vi "Color_Sensor.vi"(11 "PhoenixMotorControlDevRef":T1={"DeviceStatus"={"status"=FALSE, "code"=0, "source"=""}, "Type"=enum."PWM", "PWM"={"PWM Channel"=enum."PWM 1", "DeadBand"={"Name"="", "maxPositivePwm"=0, "minPositivePwm"=0, "centerPwm"=0, "maxNegativePwm"=0, "minNegativePwm"=0, "angularRange"=0}}, "CAN"={"Device Number"=0, "SetOutput VI Ref"=variant(enum8{"Percent VBus", "Current", "Speed", "Position", "Voltage"} enum."Percent VBus"), "GetOutput VI Ref"=variant(refnum<k1> refnum), "Enable VI Ref"=variant(dbl 12.0), "Disable VI Ref"=variant(enum8{"Percent VBus", "Speed", "Position", "Slave", "Unchanged / Invalid", "Voltage Compensation", "Current", "Motion Profile"} enum."Percent VBus"), "Data"=variant}, "Invert"=FALSE, "DIO PWM"={"PWM \"Enable\" Channel"=enum."Invalid", "DIOChannel"=enum."Invalid", "PWM Rate"=0.0}}) -> ()   [LabVIEW 2019]
uses:
  <vilib>/Rock Robotics/WPI/MotorControl/WPI_MotorControlDeviceRef.ctl
  <vilib>/Rock Robotics/WPI/MotorControl/WPI_MotorControlType.ctl
  <vilib>/Rock Robotics/SystemInterfaces/DIO/FPGA_DIOPWMChannel.ctl
  <vilib>/Rock Robotics/WPI/PWM/WPI_PWMDeadband.ctl
  <vilib>/Rock Robotics/SystemInterfaces/DIO/FPGA_DIOChannel.ctl
  <vilib>/Rock Robotics/WPI/ThirdParty/Phoenix-LabVIEW/Motor Controller/Controls/CTRE_Phoenix_MotorControl_ControlMode.ctl
panel:
  out "Color Match? 2":bool
  out "Matched Color Name 2":string
  out "Match Confidence 2":dbl
  out "Measured Color 2":cluster{"R":dbl, "G":dbl, "B":dbl}
  out "error out 2":errorcluster
  out "Proximity 2":u16(graph)
  out "Color 2":u32(colorbox)
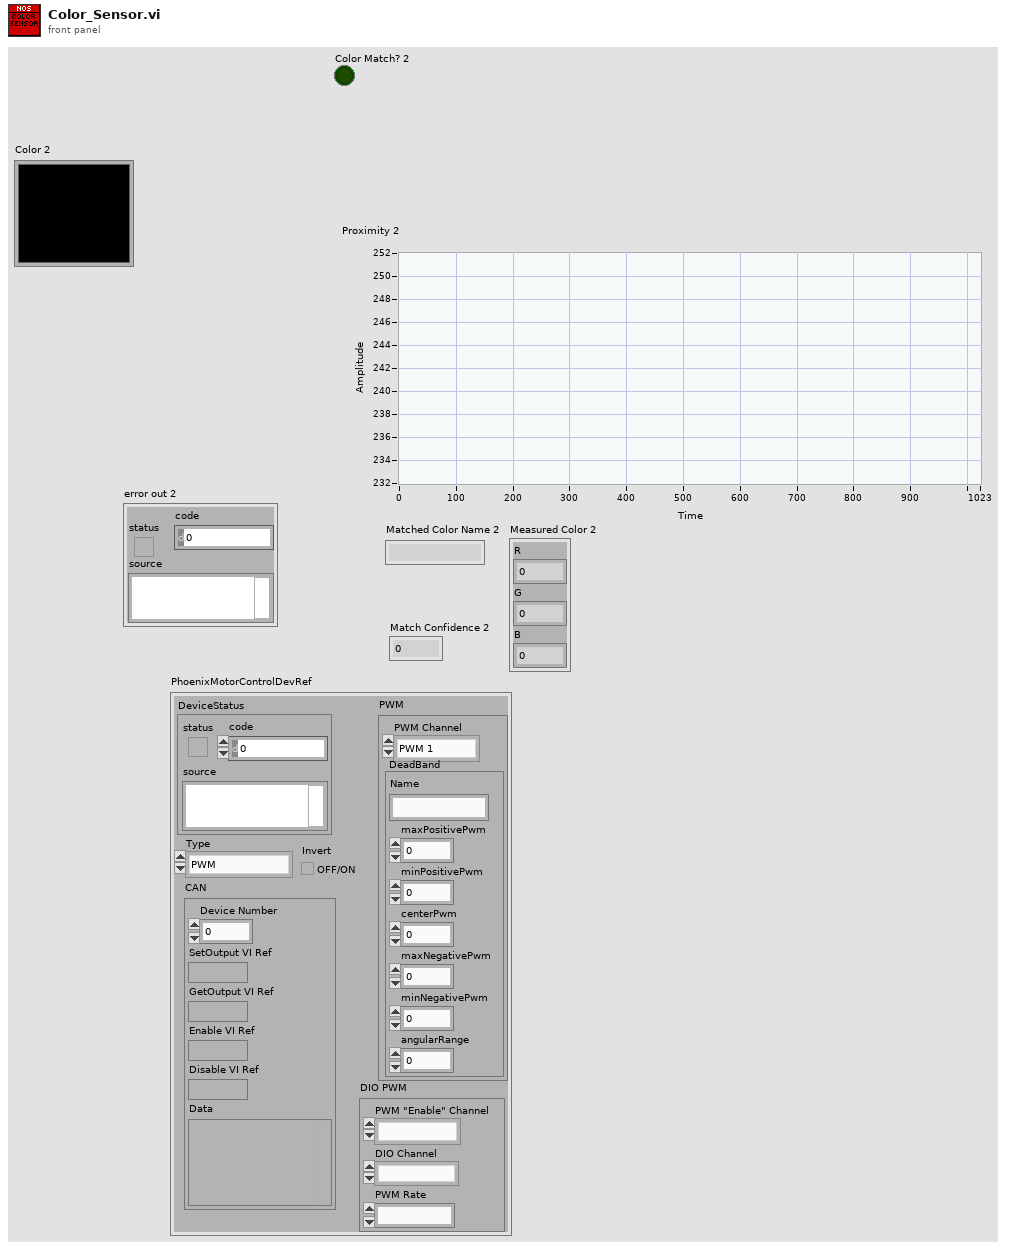
[diagram p1: front panel]
types:
  T1 = typedef "WPI_MotorControlDeviceRef.ctl" = cluster{"DeviceStatus":errorcluster, "Type":T2, "PWM":cluster{"PWM Channel":T3, "DeadBand":T4}, "CAN":cluster{"Device Number":u8, "SetOutput VI Ref":variant, "GetOutput VI Ref":variant, "Enable VI Ref":variant, "Disable VI Ref":variant, "Data":variant}, "Invert":bool, "DIO PWM":cluster{"PWM \"Enable\" Channel":T3, "DIOChannel":T5, "PWM Rate":dbl}}
  T2 = typedef "WPI_MotorControlType.ctl" = enum16{"PWM", "CAN", "DIO PWM"}
  T3 = typedef "FPGA_DIOPWMChannel.ctl" = enum8{"PWM 0", "PWM 1", "PWM 2", "PWM 3", "PWM 4", "PWM 5", "PWM 6", "PWM 7", "PWM 8", "PWM 9", "PWM MXP 0", "PWM MXP 1", "PWM MXP 2", "PWM MXP 3", "PWM MXP 4", "PWM MXP 5", "PWM MXP 6", "PWM MXP 7", "PWM MXP 8", "PWM MXP 9", "Invalid"}
  T4 = typedef "WPI_PWMDeadband.ctl" = cluster{"Name":string, "maxPositivePwm":i32, "minPositivePwm":i32, "centerPwm":i32, "maxNegativePwm":i32, "minNegativePwm":i32, "angularRange":u16}
  T5 = typedef "FPGA_DIOChannel.ctl" = enum8{"DIO 0", "DIO 1", "DIO 2", "DIO 3", "DIO 4", "DIO 5", "DIO 6", "DIO 7", "DIO 8", "DIO 9", "DIO MXP 0", "DIO MXP 1", "DIO MXP 2", "DIO MXP 3", "DIO MXP 4", "DIO MXP 5", "DIO MXP 6", "DIO MXP 7", "DIO MXP 8", "DIO MXP 9", "DIO MXP 10", "DIO MXP 11", "DIO MXP 12", "DIO MXP 13", "DIO MXP 14", "DIO MXP 15", "SPI Port CS1", "SPI Port CS2", "SPI Port CS3", "SPI Port MISO", "SPI Port MOSI", "Invalid"}
  T6 = typedef "CTRE_Phoenix_MotorControl_ControlMode.ctl" = u16
  T7 = typedef "Color Sensor V3 DevRef.ctl" = cluster{"I2CDevRef":T8}
  T8 = typedef "WPI_I2CDevRef.ctl" = cluster{"DevStatus":errorcluster, "Device Address":u8, "Handle":i32, "I2C Bus":T9}
  T9 = typedef "i2c_bus.ctl" = enum16{"I2C On-Board", "I2C MXP", "Invalid"}
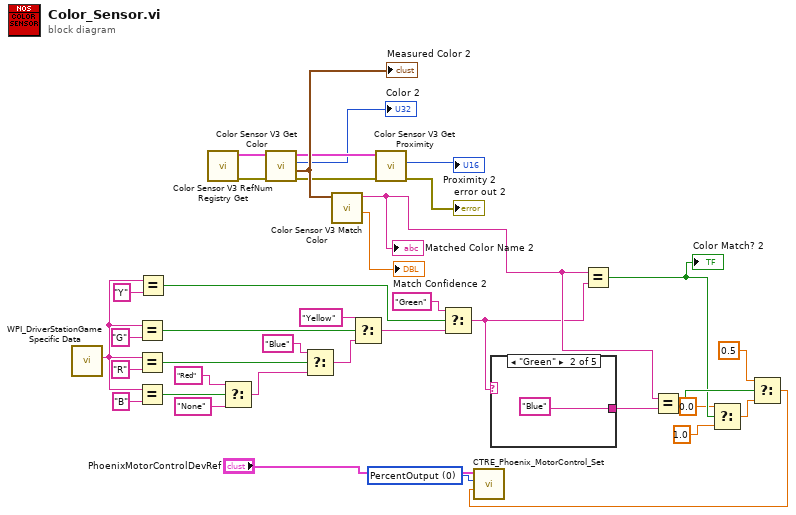
[diagram p0: block diagram]
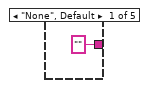
[diagram p2: hidden frame]
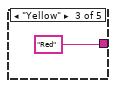
[diagram p3: hidden frame]
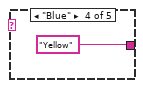
[diagram p4: hidden frame]
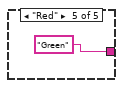
[diagram p5: hidden frame]
diagram:
  w38 = T6 0 items=["PercentOutput"=0, "Position"=1, "Velocity"=2, "Current"=3, "Follower"=5, "MotionProfile"=6, "MotionMagic"=7, "MotionProfileArc"=10, "Disabled"=15] ("Control Mode")
  n1 = call <vilib>:"WPI_DriverStationGame Specific Data.vi"() -> ("Game Specific Data"=w22:string)  [unwired: 11 in]
  n2 = Equal?(x=w22, y="G") -> (x = y?=w27:bool)
  n3 = Equal?(x=w22, y="R") -> (x = y?=w24:bool)
  n4 = Equal?(x=w22, y="B") -> (x = y?=w23:bool)
  n5 = Equal?(x=w22, y="Y") -> (x = y?=w29:bool)
  n6 = call <vilib>:"Color Sensor V3 RefNum Registry Get.vi"() -> ("error out"=w30:errorcluster, "ColorSensorDevRef"=w31:T7)  [unwired: 10 in]
  n7 = Select(t="Red" ("Color"), s=w23, f="None") -> (s? t:f=w25:string)
  n8 = call <vilib>:"Color Sensor V3 Get Color.vi"("error in (no error)"=w30, "ColorSensorDevRef"=w31) -> ("error out"=w16:errorcluster, "Normalized Color"=w20:cluster{"R":dbl, "G":dbl, "B":dbl}, "Color"=→"Color 2":u32, "ColorSensorDevRef out"=w17:T7)  [unwired: 6 in]
  "Measured Color 2" <- w20
  n9 = Select(t="Blue", s=w24, f=w25) -> (s? t:f=w26:string)
  n10 = call <vilib>:"Color Sensor V3 Match Color.vi"("Measured Color"=w20) -> ("Confidence"=→"Match Confidence 2":dbl, "Matched Color Name"=w35:string)  [unwired: 8 in, 1 out]
  "Matched Color Name 2" <- w35
  n11 = Select(t="Yellow", s=w27, f=w26) -> (s? t:f=w28:string)
  n12 = call <vilib>:"Color Sensor V3 Get Proximity.vi"("error in (no error)"=w16, "ColorSensorDevRef"=w17) -> ("error out"=→"error out 2":errorcluster, "Proximity"=→"Proximity 2":u16)  [unwired: 7 in, 1 out]
  n13 = Select(t="Green", s=w29, f=w28) -> (s? t:f=w33:string)
  n14 = case shown="\"Green\"" w33 {
    tunnel: ["" ("t") "Blue" ("t") "Red" ("t") "Yellow" ("t") "Green" ("t")] -> w34
    frame "None", Default {
    }
    frame "Green" {
    }
    frame "Yellow" {
    }
    frame "Blue" {
    }
    frame "Red" {
    }
  }
  n15 = Equal?(x=w35, y=w33) -> (x = y?=w32:bool)
  "Color Match? 2" <- w32
  n16 = Equal?(x=w35, y=w34) -> (x = y?=w37:bool)
  n17 = Select(t=0.0, s=w32, f=1.0 ("Output")) -> (s? t:f=w36:dbl)
  n18 = Select(t=0.5, s=w37, f=w36) -> (s? t:f=w2:dbl)
  n19 = call <vilib>:"CTRE_Phoenix_MotorControl_Set.vi"("Output"=w2, "Control Mode"=w38, "PhoenixMotorControlDevRef"="PhoenixMotorControlDevRef") -> ()  [unwired: 7 in, 2 out]
